vi "xyImageKoordinates.vi"(8 "error in (no error)":errorcluster, 11 "String":string="pike.calibration=\"0,-0.00387,0,0.003225;1376,0.0050052,0,0.003225;0,-0.00387,1040,-0.003483\"\npike.scan=\"0,0,10,0.00119;0,0,3,-7.2266666667E-5;0,0,4,-8.8133333333E-5;0,0,11,0;0,0,12,0;0,0,7,3;0,4,9,127;0,2,3,0.05875;0,2,4,0;0,2,11,100000;0.00255,2,11,0;0.00256,1,12,1;0.00256,0,7,1;0.00256,2,3,-1.4928955695E-16;0.00256,2,4,0.0073046875;0.00264,0,7,3;0.00264,2,3,-0.05875;0.00264,2,4,0;0.00264,2,11,-100000;0.00519,2,11,0;0.0052,1,12,1;0.0052,0,7,1;0.0052,2,3,1.4928955695E-16;0.0052,2,4,0.0073046875;0.00528,0,7,3;0.00528,5,9,0;0.67056,2,3,0.05875;0.67056,2,4,0;0.67056,2,11,100000;0.67311,2,11,0;0.67312,1,12,1;0.67312,0,7,1;0.67312,2,3,-1.4928955695E-16;0.67312,2,4,0.0073046875;0.6732,0,7,3;0.6732,2,3,-0.05875;0.6732,2,4,0;0.6732,2,11,-100000;0.67575,2,11,0;0.67576,2,3,0;0.67576,2,4,0;0.67576,0,7,0;\"\nstage.x=\"12\"\nstage.y=\"45\"\nobj.mag=\"10\"") -> (0 "error out":errorcluster, 1 "pixels":cluster{"xpixel":i32, "yPixel":i32}, 2 "fast/slow [m(ii)]":cluster{"x":dbl, "y":dbl}[](array[cluster]), 3 "start [m(ii)] (without stage)":cluster{dbl, dbl}, 4 "stage [m]":cluster{dbl, dbl}, 6 "used magnification":sgl)   [LabVIEW 2011]
panel:
  out "calibrated":bool
  # "first search for calibration, then check for scan"
  # "for scan we need"
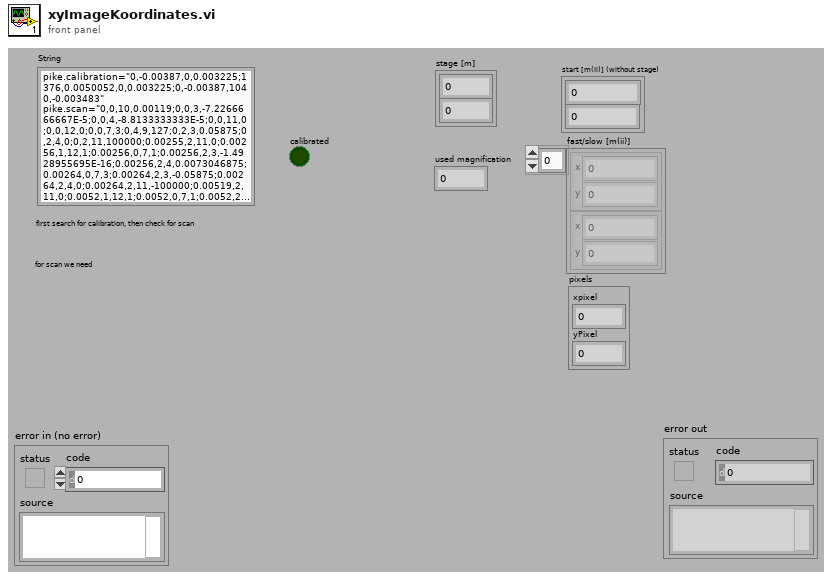
[diagram p1: front panel]
types:
  T1 = typedef "ScanControl.ctl" = cluster{"Time [s]":dbl, "action":T2, "channel":T3, "value (/s)":dbl}[]
  T2 = typedef "ScanControl_Action.ctl" = enum16{"Abs", "Rel", "Inc", "IncInc", "LoopStart", "LoopEnd", "WaitTriggerRising"}
  T3 = typedef "ScanControl_Channel.ctl" = enum16{"Com", "AnalogConfig", "AnalogValue", "GalvoX", "GalvoY", "Galvo3", "Galvo4", "Digital", "Free", "Loop", "SMoveTime", "Image1X", "Image1Y", "Image2X", "Image2Y"}
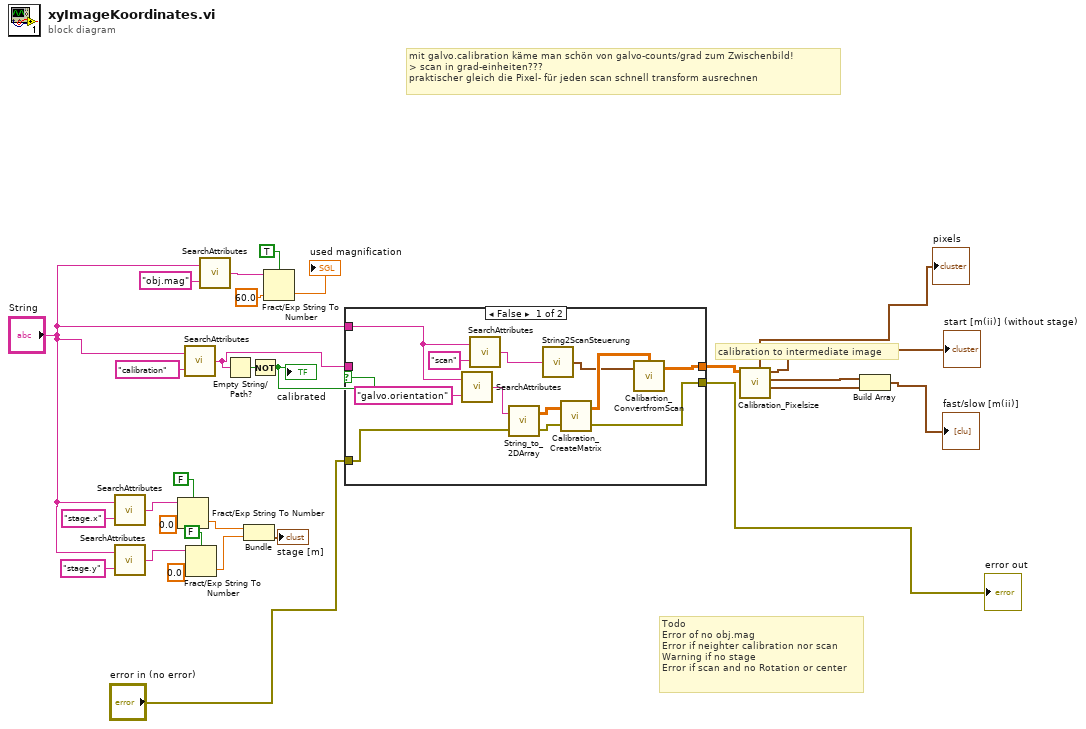
[diagram p0: block diagram]
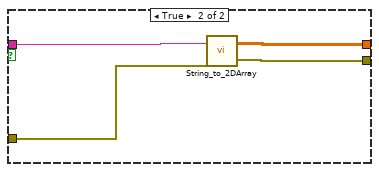
[diagram p2: hidden frame]
diagram:
  # "calibration to intermediate image"
  # "Todo\nError of no obj.mag\nError if neighter calibration nor scan\nWarning if no stage\nError if scan and no Rotation or center"
  # "mit galvo.calibration käme man schön von galvo-counts/grad zum Zwischenbild!\n> scan in grad-einheiten???\npraktischer gleich die Pixel- für jeden scan schnell transform ausrechnen"
  n1 = call "SearchAttributes.vi"("Search"="stage.x", "String"="String") -> ("ValueText"=w17:string)
  n2 = call "SearchAttributes.vi"("Search"="stage.y", "String"="String") -> ("ValueText"=w16:string)
  n3 = Fract/Exp String To Number(use system decimal point (T)=FALSE, string=w17, default (0 dbl)=0.0 ("default (0 DBL)")) -> (number=w15:dbl)  [unwired: 2 out]
  n4 = call "SearchAttributes.vi"("Search"="calibration", "String"="String") -> ("ValueText"=w28:string)
  n5 = Fract/Exp String To Number(use system decimal point (T)=FALSE, string=w16, default (0 dbl)=0.0 ("default (0 DBL)")) -> (number=w14:dbl)  [unwired: 2 out]
  n6 = call "SearchAttributes.vi"("Search"="obj.mag", "String"="String") -> ("ValueText"=w12:string)
  n7 = Empty String/Path?(string/path=w28) -> (empty?=w27:bool)
  n8 = Bundle(w15, w14) -> (→"stage [m]":cluster{dbl, dbl})  [unwired: 1 out]
  n9 = Not(x=w27) -> (.not. x?=w2:bool)
  "calibrated" <- w2
  n10 = Fract/Exp String To Number(use system decimal point (T)=TRUE, string=w12, default (0 dbl)=sgl 60.0 ("default (0 DBL)")) -> (number=→"used magnification":sgl)  [unwired: 2 out]
  n11 = case shown="False" w2 {
    tunnel: w28 -> [_ w45]
    tunnel: "error in (no error)" -> [w32 w44]
    tunnel: [w30 w43] -> w6
    tunnel: [w41 w42] -> w5
    tunnel: "String" -> [w38 _]
    frame False {
      n12 = call "SearchAttributes.vi"("Search"="galvo.orientation", "String"=w38) -> ("ValueText"=w37:string)
      n13 = call "SearchAttributes.vi"("Search"="scan", "String"=w38) -> ("ValueText"=w34:string)
      n14 = call "String_to_2DArray.vi"("error in (no error)"=w32, "String"=w37) -> ("error out"=w31:errorcluster, "Array"=w36:dbl[][])  [unwired: 2 in]
      n15 = call "String2ScanSteuerung.vi"("String"=w34) -> ("ScanSteuerung"=w33:T1)
      n16 = call "Calibration_CreateMatrix.vi"("error in (no error)"=w31, "CalibrationCoordinates: x,x',y,y'..."=w36) -> ("error out"=w30:errorcluster, "Linear conversion Matrix"=w35:dbl[][])
      n17 = call "Calibartion_ConvertfromScan.vi"("ScanSteuerung"=w33, "Linear conversion Matrix"=w35) -> ("calibartion [m]"=w41:dbl[][])  [unwired: 2 in]
    }
    frame True {
      n18 = call "String_to_2DArray.vi"("error in (no error)"=w44, "String"=w45) -> ("error out"=w43:errorcluster, "Array"=w42:dbl[][])  [unwired: 2 in]
    }
  }
  "error out" <- w6
  n19 = call "Calibration_Pixelsize.vi"("CalibrationCoordinates: x,x'y,y'..."=w5) -> ("slow"=w3:cluster{"x'":dbl, "y'":dbl}, "Fast"=w4:cluster{"x'":dbl, "y'":dbl}, "Start"=→"start [m(ii)] (without stage)":cluster{"x'":dbl, "y'":dbl}, "Pixels"=→"pixels":cluster{u32, u32})  [unwired: 7 out]
  n20 = Build Array(w4, w3) -> (→"fast/slow [m(ii)]":cluster{"x'":dbl, "y'":dbl}[])
